vi "VsEPCal-Adjust Shaker Amp.vi"(10 "Hidden":T2={"AO Sampling Rate (Hz)"=100000.0, "AI Sampling Rate (Hz)"=100000.0, "Masker Timing"={"Active"=FALSE, "Delay (ms)"=0.0, "Width (ms)"=0.0, "Ramp (ms)"=0.0}, "Jerk rise time (ms)"=2.0, "Masker atten"=0.0, "show adjust"=FALSE, "linear gain"=FALSE}, 11 "Stimulus":T1={"Rep rate (Hz)"=20.0, "Start (dB atten)"=60.0, "Stop (dB atten)"=10.0, "Step (dB)"=10.0}) -> ()   [LabVIEW 2020]
uses:
  Typedefs/VsEP-Hidden Params.ctl
  epl-vi-lib/Signal Synthesis VIs/Controls/Gate XCtl/Gate Control.xctl
  Typedefs/VsEPCal- Stimulus.ctl
  epl-vi-lib/Connection VIs/Type Defs/Output sources.ctl
  epl-vi-lib/Connection VIs/Type Defs/Input sources.ctl
  epl-vi-lib/PXI DAQ VIs/DAQ Engine VIs/PXI Globals.vi
panel:
  out "Graph":dbl[][](graph)
  out "Abort":bool
  in  "START":bool
  in  "RETURN":bool
  in  "STOP":bool
  # "1. Disconnect shaker from Crown amplifier.\n\n2. Monitor Crown output on oscilloscope and/or connect Crown \noutput to Accelerometer input to monitor on graph below. \n\n3. Press Start\n\n4. Adjust gain of Crown amplifier to make signal amplitude 5V.\n\n5. Stop\n\n6. Reconnect shaker to Crown amplifier.\n\n7. Return"
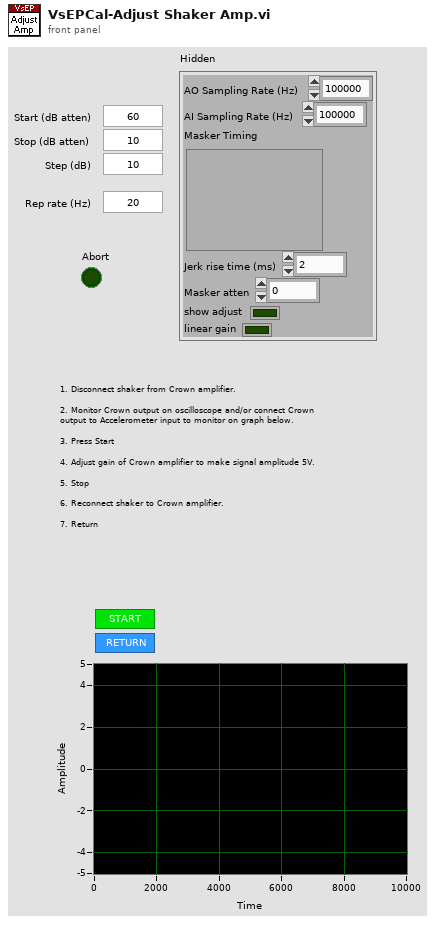
[diagram p1: front panel]
types:
  T1 = typedef "VsEPCal- Stimulus.ctl" = cluster{"Rep rate (Hz)":dbl, "Start (dB atten)":dbl, "Stop (dB atten)":dbl, "Step (dB)":dbl}
  T2 = typedef "VsEP-Hidden Params.ctl" = cluster{"AO Sampling Rate (Hz)":dbl, "AI Sampling Rate (Hz)":dbl, "Masker Timing":cluster{"Active":bool, "Delay (ms)":dbl, "Width (ms)":dbl, "Ramp (ms)":dbl}, "Jerk rise time (ms)":dbl, "Masker atten":dbl, "show adjust":bool, "linear gain":bool}
  T3 = typedef "Input sources.ctl" = u16
  T4 = typedef "Output sources.ctl" = u16
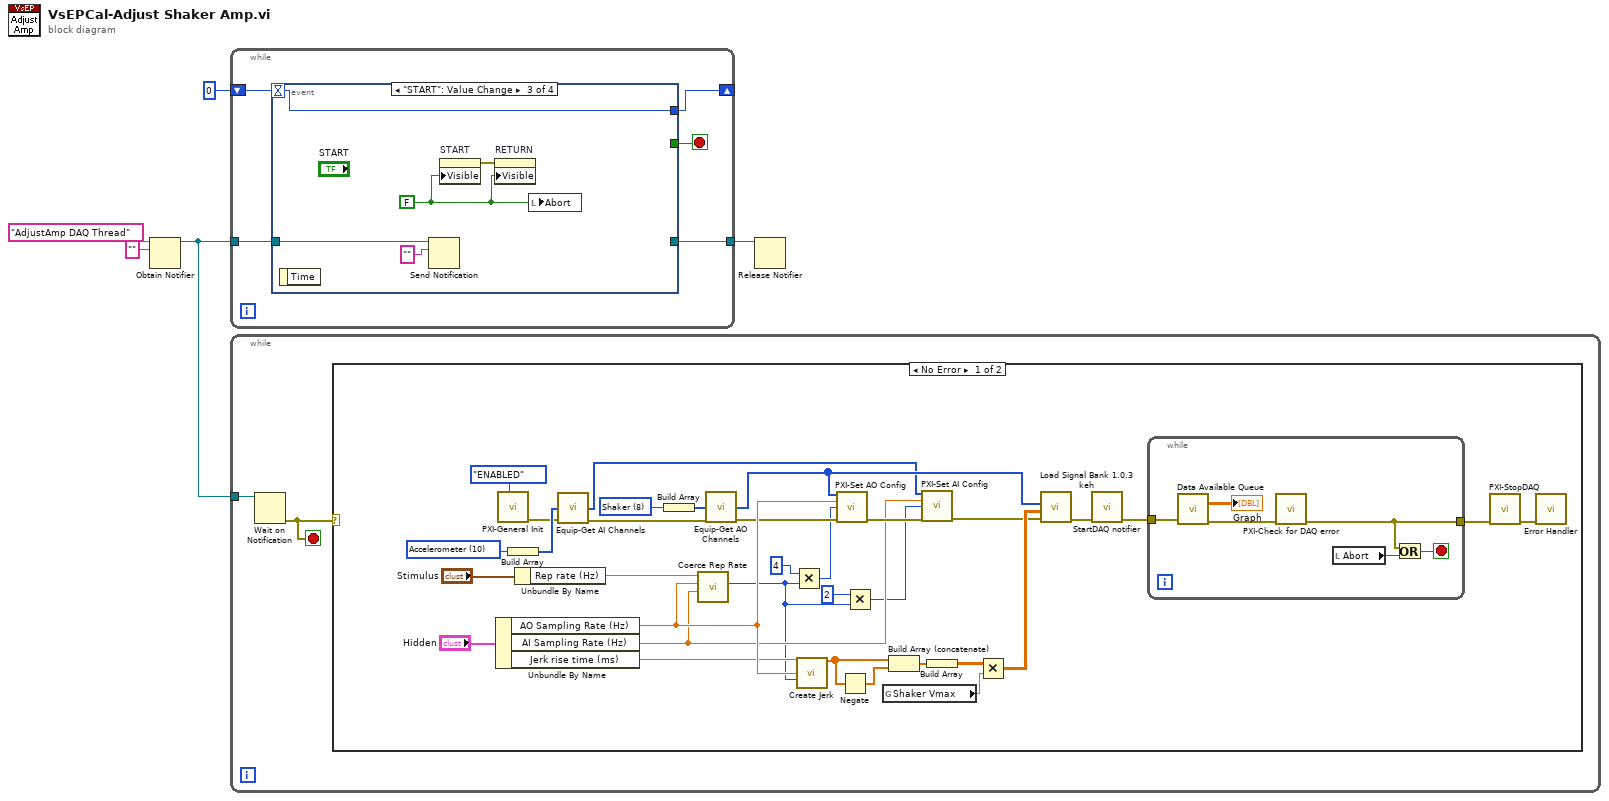
[diagram p0: block diagram]
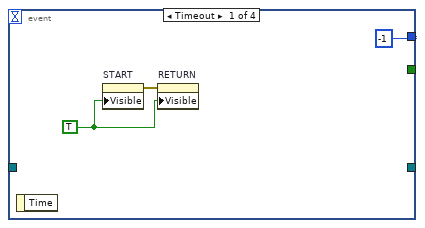
[diagram p3: hidden frame]
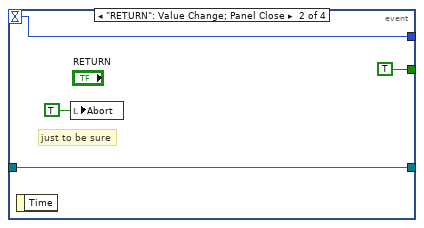
[diagram p4: hidden frame]
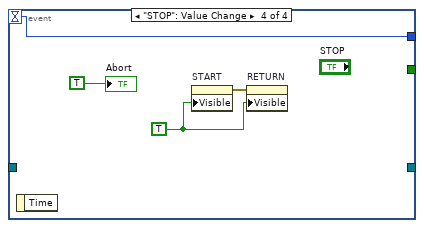
[diagram p5: hidden frame]
diagram:
  n1 = Obtain Notifier(name (unnamed)="AdjustAmp DAQ Thread", notification data type="") -> (notifier out=w4:refnum<notifier>)  [unwired: 2 in, 2 out]
  n2 = while {
    tunnel: w4 -> [w9]
    tunnel: [w8] -> w5
    shift-right: [w6] -> _
    shift-left: 0 -> [w7]
    stop <- w10 stop-if-true
    n3 = event shown="[2] \"START\": Value Change" {
      selector: _ -> [_ _ _ _]
      dyn-events: _ -> [_ _ _ _]
      timeout: w7 -> [_ w14 w19 w23]
      tunnel: [_ TRUE _ _] -> w10
      tunnel: w9 -> [_ w16 w21 _]
      tunnel: [_ w16 _ _] -> w8
      tunnel: [-1 w14 w19 w23] -> w6
      event Timeout {
        w12 = TRUE
        n4 = event-data() -> ()  [unwired: 1 in, 1 out]
        n5 = property on="START" class="Bool"("Visible"=w12) -> (error out=w13:errorcluster)  [unwired: 2 in, 1 out]
        n6 = property on="RETURN" class="Bool"(error in=w13, "Visible"=w12) -> ()  [unwired: 1 in, 2 out]
      }
      event "RETURN": Value Change; Panel Close {
        # "just to be sure"
        n7 = event-data() -> ()  [unwired: 1 in, 1 out]
        n8 = local write "Abort"(TRUE ("Abort")) -> ()
      }
      event "START": Value Change {
        w18 = FALSE
        n9 = event-data() -> ()  [unwired: 1 in, 1 out]
        n10 = Send Notification(notification="", notifier=w21) -> ()  [unwired: 1 in, 2 out]
        n11 = property on="START" class="Bool"("Visible"=w18) -> (error out=w22:errorcluster)  [unwired: 2 in, 1 out]
        n12 = property on="RETURN" class="Bool"(error in=w22, "Visible"=w18) -> ()  [unwired: 1 in, 2 out]
        n13 = local write "Abort"(w18) -> ()
      }
      event "STOP": Value Change {
        w25 = TRUE
        n14 = event-data() -> ()  [unwired: 1 in, 1 out]
        n15 = property on="START" class="Bool"("Visible"=w25) -> (error out=w26:errorcluster)  [unwired: 2 in, 1 out]
        n16 = property on="RETURN" class="Bool"(error in=w26, "Visible"=w25) -> ()  [unwired: 1 in, 2 out]
        "Abort" <- TRUE
      }
    }
  }
  n17 = while {
    tunnel: w4 -> [w28]
    stop <- w27 stop-if-true
    n18 = Wait on Notification(notifier=w28) -> (error out=w27:errorcluster)  [unwired: 3 in, 3 out]
    n19 = case shown="No Error" w27 {
      frame No Error {
        w39 = T3 10 items=["--unused--", "Probe Mic Right", "Probe Mic Left", "Cal Mic", "ABR", "CAP Right", "CAP Left", "Startle piezo", "Temperature", "Heart rate", "Accelerometer"] ("Ring")
        w56 = T4 8 items=["--unused--", "Right primary", "Right secondary", "Left primary", "Left secondary", "Shocks", "Startle", "Background", "Shaker"] ("Ring")
        n20 = Unbundle By Name("Hidden") -> ("AO Sampling Rate (Hz)"=w61:dbl, "AI Sampling Rate (Hz)"=w33:dbl, "Jerk rise time (ms)"=w50:dbl)
        n21 = call "PXI-General Init.vi"("Double Buffer Mode"=enum32{"OFF", "ENABLED", "FORCED"}."ENABLED") -> ("error out"=w38:errorcluster)  [unwired: 10 in]
        n22 = Build Array(w39) -> (w40:T3[])
        n23 = Unbundle By Name("Stimulus") -> ("Rep rate (Hz)"=w51:dbl)
        n24 = call "Equip-Get AI Channels.vi"("Inputs"=w40, "error in (no error)"=w38) -> ("AI Channels"=w34:i32[], "error out"=w37:errorcluster)  [unwired: 12 in]
        n25 = Build Array(w56) -> (w57:T4[])
        n26 = call "Coerce Rep Rate.vi"("AI sampling rate (Hz)"=w33, "AO sampling rate (Hz)"=w61, "Rep rate (Hz)"=w51) -> ("AO npts"=w31:i32)  [unwired: 5 in, 3 out]
        n27 = call "Equip-Get AO Channels.vi"("Outputs"=w57, "error in (no error)"=w37) -> ("AO Channels"=w52:i32[], "error out"=w54:errorcluster)  [unwired: 12 in]
        n28 = Multiply(x=4, y=w31) -> (x*y=w32:i32)
        n29 = call "Create Jerk.vi"("Rise time (ms)"=w50, "Sampling Rate (Hz)"=w61, "Npts"=w31) -> ("Waveform"=w49:dbl[])  [unwired: 11 in, 1 out]
        n30 = call "PXI-Set AO Config.vi"("AO Channels"=w52, "Sampling Rate (Hz)"=w61, "Buffer Size"=w32, "error in (no error)"=w54) -> ("error out"=w36:errorcluster)  [unwired: 11 in]
        n31 = Negate(x=w49) -> (-x=w48:dbl[])
        n32 = Multiply(x=2, y=w31) -> (x*y=w29:i32)
        n33 = global read "PXI Globals.vi" "Shaker Vmax"() -> (w45:dbl)
        n34 = Build Array (concatenate)(w49, w48) -> (w47:dbl[])
        n35 = call "PXI-Set AI Config.vi"("AI Channels"=w34, "Sampling Rate (Hz)"=w33, "Buffer Size"=w29, "error in (no error)"=w36) -> ("error out"=w35:errorcluster)  [unwired: 11 in]
        n36 = Build Array(w47) -> (w46:dbl[][])
        n37 = Multiply(x=w46, y=w45) -> (x*y=w44:dbl[][])
        n38 = call "Load Signal Bank 1.0.3 keh.vi"("error in (no error)"=w35, "Input array"=w44, "Active AO Array"=w52) -> ("error out"=w55:errorcluster)  [unwired: 6 in, 2 out]
        n39 = call "StartDAQ notifier.vi"("error in (no error)"=w55) -> ("error out"=w42:errorcluster)  [unwired: 6 in]
        n40 = while {
          tunnel: w42 -> [w67]
          tunnel: [w62] -> w43
          stop <- w63 stop-if-true
          n41 = call "Data Available Queue.vi"("error in (no error)"=w67) -> ("Waveform Graph"=→"Graph":dbl[][], "error out"=w64:errorcluster)  [unwired: 10 in, 3 out]
          n42 = call "PXI-Check for DAQ error.vi"("error in (no error)"=w64) -> ("error out"=w62:errorcluster)  [unwired: 14 in]
          n43 = local read "Abort"() -> (w65:bool)
          n44 = Or(x=w62, y=w65) -> (x .or. y?=w63:bool)
        }
        n45 = call "PXI-StopDAQ.vi"("error in (no error)"=w43) -> ("error out"=w41:errorcluster)  [unwired: 6 in]
        n46 = call "Error Handler.vi"("error in (no error)"=w41) -> ()  [unwired: 13 in, 2 out]
      }
      frame Error {
      }
    }
  }
  n47 = Release Notifier(notifier=w5) -> ()  [unwired: 2 in, 3 out]
